vi "Read Object Dependencies.vi"(10 "Error In":errorcluster, 11 "Dependency .NET Ref In":refnum<k24>) -> (2 "Error Out":errorcluster, 3 "Dependency Properties":T1)   [LabVIEW 2015, in "VeriStand Custom Device XML Parser.lvlib"]
doc: "Reads the properties of a dependency object"
uses:
  VeriStand Custom Device XML Parser.lvlib
  XML Controls/Dependency Properties.ctl
  NationalInstruments.VeriStand.XMLReader
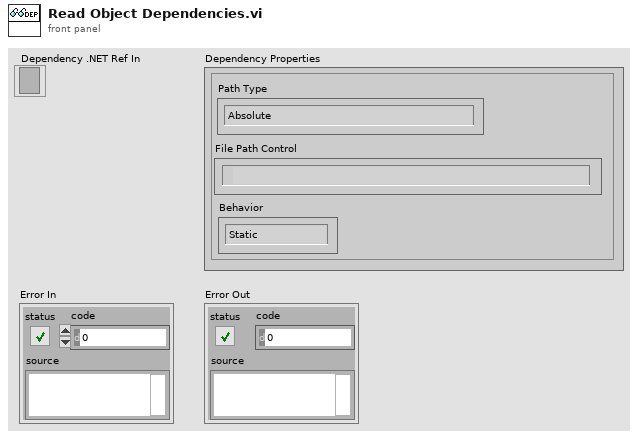
[diagram p1: front panel]
types:
  T1 = typedef "VeriStand Custom Device XML Parser.lvlib/Dependency Properties.ctl" = cluster{"File Path Control":path, "Path Type":enum16{"Absolute", "To Base", "To Common Doc Dir", "To Application Data Dir"}, "Behavior":enum16{"Static", "Dynamic"}}
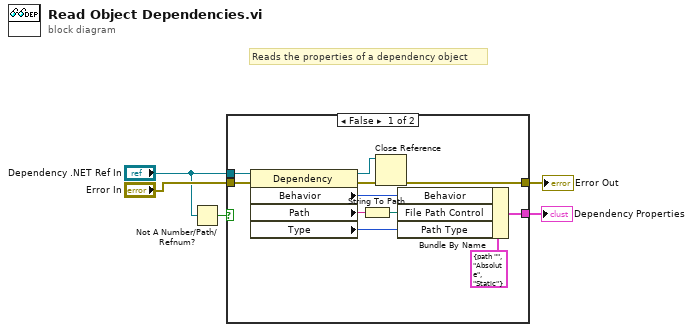
[diagram p0: block diagram]
diagram:
  # "Reads the properties of a dependency object"
  n1 = Not A Number/Path/Refnum?(number/path/refnum="Dependency .NET Ref In") -> (NaN/Path/Refnum?=w1:bool)
  n2 = case shown="False" w1 {
    tunnel: "Error In" -> [w16 w17]
    tunnel: "Dependency .NET Ref In" -> [w15 _]
    tunnel: [w7 _] -> w5
    tunnel: [w6 w17] -> w4
    frame False {
      n3 = property class="Dependency"(reference=w15, error in=w16) -> (reference out=w13:refnum<k24>, error out=w14:errorcluster, "Behavior"=w11:i32, "Path"=w8:string, "Type"=w10:i32)
      n4 = String To Path(string=w8) -> (path=w9:path)
      n5 = Close Reference(reference=w13, error in (no error)=w14) -> (error out=w6:errorcluster)
      n6 = Bundle By Name(cluster=T1 {"File Path Control"=path "", "Path Type"=enum."Absolute", "Behavior"=enum."Static"} ("Dependency"), "Behavior"=w11, "File Path Control"=w9, "Path Type"=w10) -> (w7:T1)
    }
    frame True {
    }
  }
  "Dependency Properties" <- w5
  "Error Out" <- w4
